vi "总磷启动(子VI).vi"(11 "参数":T1) -> ()   [LabVIEW 2016]
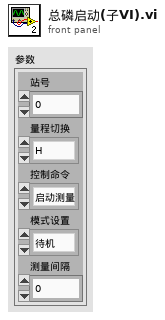
[diagram p1: front panel]
types:
  T1 = cluster{"站号":u16, "量程切换":enum32{"H", "L", "AUTO"}, "控制命令":enum16{"启动测量", "标样核查", "零点核查", "跨度核查", "空白测试", "平行样测试", "加标回收", "空白校准", "标样校准", "初始化（清洗）", "停止测试", "仪器重启", "校时", "模式设置", "测量间隔设置"}, "模式设置":enum16{"待机", "连续模式", "周期模式", "定点模式", "受控模式", "手动模式"}, "测量间隔":u16}
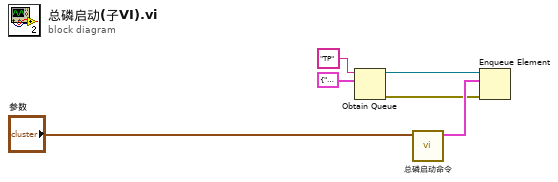
[diagram p0: block diagram]
diagram:
  n1 = Obtain Queue(name (unnamed)="TP" ("名称（未命名）"), element data type=cluster{"命令":string, "data":variant} {"命令"="", "data"=variant}) -> (queue out=w3:refnum<queue>, error out=w4:errorcluster)  [unwired: 3 in, 1 out]
  n2 = call "总磷启动命令.vi"("参数"="参数") -> ("启动命令"=w6:cluster{"命令":string, "data":variant})  [unwired: 10 in]
  n3 = Enqueue Element(queue=w3, element=w6, error in (no error)=w4) -> ()  [unwired: 1 in, 3 out]
